vi "OAT Extract Slow Roll Vectors.vi"   [LabVIEW 2017]
doc: "Extract the vectors of the specified orders from the slow roll vibration signals. The vectors are used for proximity probe signals to perform run out compensation."
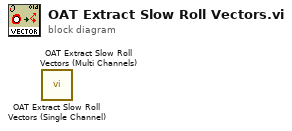
[diagram p0: block diagram]
diagram:
  n1 = call <vilib>:"OAT Extract Slow Roll Vectors (Single Channel).vi"() -> ()  [unwired: 10 in, 2 out]
  n2 = call <vilib>:"OAT Extract Slow Roll Vectors (Multi Channels).vi"() -> ()  [unwired: 10 in, 2 out]
